vi "Flash LED.vi"(4 "error in":errorcluster, 7 "Bool Refnum":refnum<vi>) -> (0 "error out":errorcluster)   [LabVIEW 2014]
doc: "This VI is a subVI for an exercise in the LabVIEW Core 3 course."
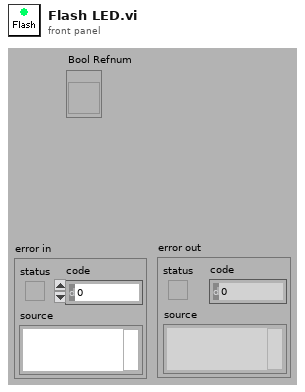
[diagram p1: front panel]
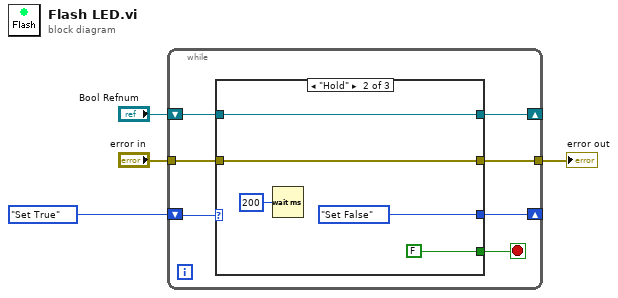
[diagram p0: block diagram]
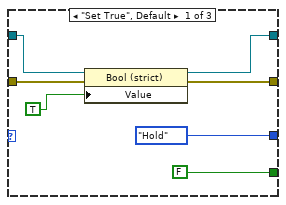
[diagram p2: hidden frame]
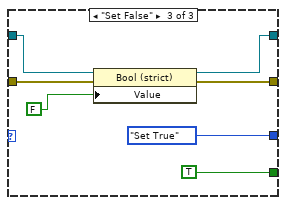
[diagram p3: hidden frame]
diagram:
  n1 = while {
    shift-right: [w10] -> _
    shift-left: "Bool Refnum" -> [w11]
    shift-right: [w7] -> _
    shift-left: enum16{"Set True", "Hold", "Set False"}."Set True" -> [w8]
    tunnel: "error in" -> [w6]
    tunnel: [w5] -> w2
    stop <- w9 stop-if-true
    n2 = case shown="\"Hold\"" w8 {
      tunnel: w11 -> [w18 w23 w30]
      tunnel: [w17 w23 w29] -> w10
      tunnel: [FALSE FALSE TRUE] -> w9
      tunnel: [enum16{"Set True", "Hold", "Set False"}."Hold" enum16{"Set True", "Hold", "Set False"}."Set False" enum16{"Set True", "Hold", "Set False"}."Set True"] -> w7
      tunnel: w6 -> [w12 w19 w26]
      tunnel: [w13 w19 w25] -> w5
      frame "Set True", Default {
        n3 = property class="Bool (strict)"(reference=w18, error in=w12, "Value"=TRUE) -> (reference out=w17:refnum<vi>, error out=w13:errorcluster)
      }
      frame "Hold" {
        n4 = Wait (ms)(milliseconds to wait=u32 200 ("millisecond multiple")) -> ()  [unwired: 1 out]
      }
      frame "Set False" {
        n5 = property class="Bool (strict)"(reference=w30, error in=w26, "Value"=FALSE) -> (reference out=w29:refnum<vi>, error out=w25:errorcluster)
      }
    }
  }
  "error out" <- w2
